vi "_Parse DBL Array Result.vi"(8 "error in (no error)":errorcluster, 10 "Input String":string, 11 "VISA resource name":refnum<visa-resource-name>) -> (0 "error out":errorcluster, 1 "Results":dbl[](array[numeric]) format="%^.3e", 2 "Reliability":i32, 3 "VISA resource name out":refnum<visa-resource-name>)   [LabVIEW 2020, in "Rohde&Schwarz CMP LR WPAN Measurement.lvlib"]
uses:
  <instrlib>/Rohde&Schwarz CMP LR WPAN Measurement/Rohde&Schwarz CMP LR WPAN Measurement.lvlib
  <instrlib>/Rohde&Schwarz CMP LR WPAN Measurement/Private/rsidr_core.llb/rsidr_core.lvlib
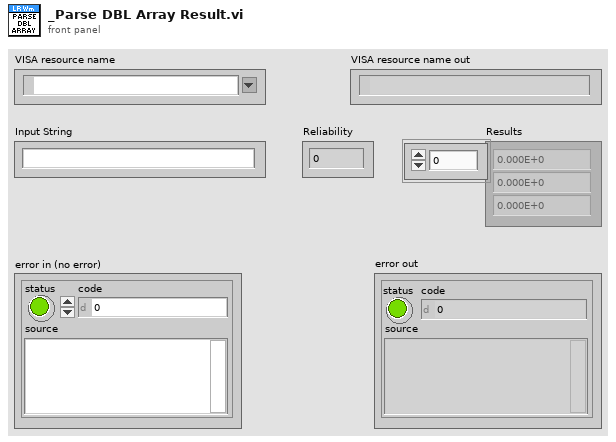
[diagram p1: front panel]
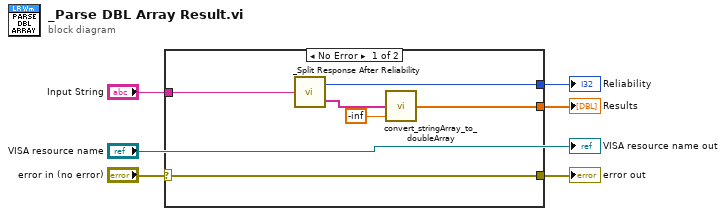
[diagram p0: block diagram]
diagram:
  n1 = case shown="No Error" "error in (no error)" {
    selector: "error in (no error)" -> [w8 w13]
    tunnel: [w11 _] -> w5
    tunnel: [w10 _] -> w4
    tunnel: "Input String" -> [w9 _]
    tunnel: [w8 w13] -> w2
    frame No Error {
      n2 = call <instrlib>:"_Split Response After Reliability.vi"("Input String"=w9) -> ("Response out"=w12:string[], "Reliability out"=w11:i32)
      n3 = call <instrlib>:"convert_stringArray_to_doubleArray.vi"("default (0)"=-inf ("Negative Infinity"), "string array in"=w12) -> ("double array out"=w10:dbl[])  [unwired: 3 in]
    }
    frame Error {
    }
  }
  "error out" <- w2
  "Reliability" <- w5
  "Results" <- w4
  "VISA resource name out" <- "VISA resource name"
